vi "Draw Dot.vi"(6 "Color":u32(colorbox)=16711680, 7 "CenterX":sgl, 8 "error in (no error)":errorcluster, 9 "Size":sgl=7.0, 10 "CenterY":sgl, 11 "Refnum in":T1) -> (0 "error out":errorcluster, 3 "Refnum out":T1)   [LabVIEW 2012]
uses:
  <vilib>/vision/Image Controls.llb/IMAQ Image.ctl
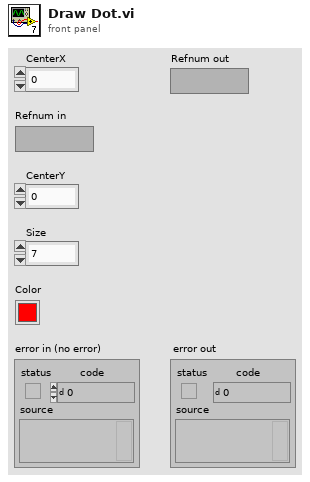
[diagram p1: front panel]
types:
  T1 = typedef "IMAQ Image.ctl" = refnum<image>
  T2 = cluster{"Left":i32, "Top":i32, "Right":i32, "Bottom":i32}
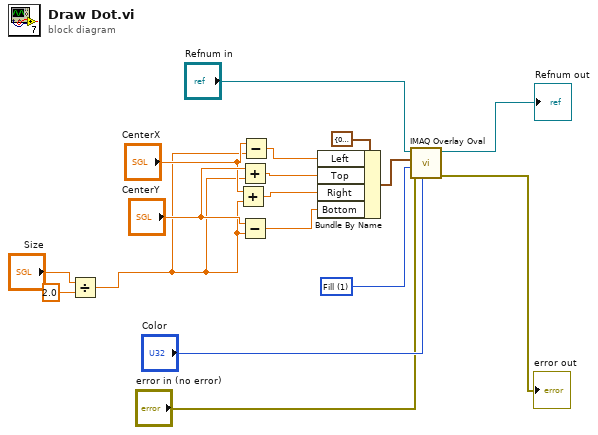
[diagram p0: block diagram]
diagram:
  w16 = u32 1 items=["Frame", "Fill"] ("Drawing Mode (Frame)")
  n1 = Divide(x="Size", y=2.0) -> (x/y=w1:dbl)
  n2 = Add(x="CenterX", y=w1) -> (x+y=w9:dbl)
  n3 = Add(x="CenterY", y=w1) -> (x+y=w6:dbl)
  n4 = Subtract(x="CenterY", y=w1) -> (x-y=w10:dbl)
  n5 = Subtract(x="CenterX", y=w1) -> (x-y=w8:dbl)
  n6 = Bundle By Name(cluster=T2 {"Left"=0, "Top"=0, "Right"=0, "Bottom"=0} ("Bounding Rectangle"), "Left"=w8, "Top"=w6, "Right"=w9, "Bottom"=w10) -> (w5:T2)
  n7 = call "IMAQ Overlay Oval"("Color"="Color", "error in (no error)"="error in (no error)", "Drawing Mode (Frame)"=w16, "Bounding Rectangle"=w5, "Image"="Refnum in") -> ("error out"=→"error out":errorcluster, "Image Out"=→"Refnum out":T1)  [unwired: 5 in]
